vi "New Transceiver Interface.vi"(5 "FIFO Debug Flags":refnum<class "FIFO Flags.lvclass">, 7 "fifo depths (10)":u32=10, 8 "error in (no error)":errorcluster, 10 "error size (512 B)":T1=enum."512-byte", 11 "Transceiver Interface type":refnum<class "Transceiver Interface.lvclass">) -> (0 "error out":errorcluster, 3 "Transceiver Interface":refnum<class "Transceiver Interface.lvclass">)   [LabVIEW 2017, in "DSF Core.lvlib" / "Transceiver Interface.lvclass"]
uses:
  Transceiver Interface.lvclass
  C:/github/data-sharing-framework/Data Sharing Framework/Source/Core/Engine/Classes/Interface/Interface.lvclass
  Interface/Error Queue Sizes.ctl
  Debug/FIFO Flags/FIFO Flags.lvclass
  Interface/Interface.lvclass
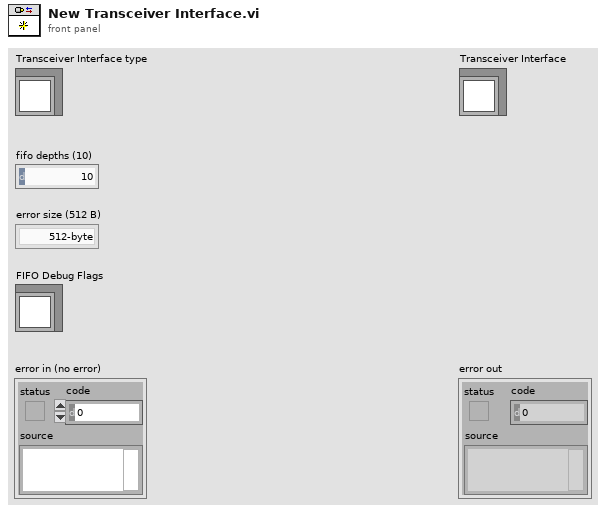
[diagram p1: front panel]
types:
  T1 = typedef "DSF Core.lvlib/Interface.lvclass/Error Queue Sizes.ctl" = enum16{"256-byte", "512-byte", "1024-byte"}
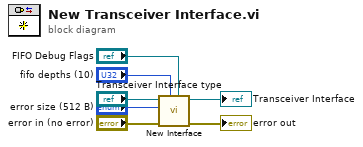
[diagram p0: block diagram]
diagram:
  n1 = call "New Interface.vi"("FIFO Debug Flags"="FIFO Debug Flags", "fifo/queue depths (10)"="fifo depths (10)", "error in (no error)"="error in (no error)", "error size (512 B)"="error size (512 B)", "Interface type"="Transceiver Interface type") -> ("error out"=→"error out":errorcluster, "Interface"=→"Transceiver Interface":refnum<class "Transceiver Interface.lvclass">)  [unwired: 5 in]
